vi "PointGrey Grasshopper_Settings.vi"(9 "Which cameras record":bool[](array[boolean]), 10 "Camera to address":i32 min=0 max=0 step=1, 11 "Camera References":T1[](array[typedef])) -> (1 "Which cameras record out":bool[](array[boolean]))   [LabVIEW 2015]
uses:
  <vilib>/userdefined/High Color/IMAQdx.ctl
  <vilib>/vision/driver/IMAQdx.llb/IMAQdx Attribute Visibility.ctl
  <vilib>/Utility/miscctls.llb/LVOutOfRangeActionTypeDef.ctl
  <vilib>/vision/driver/NI_Vision_Acquisition_Software.lvlib
  <resource>/objmgr/imaqdx.rc
panel:
  in  "CameraCommand":string
  in  "CameraEnum":u16(ring) items=["Off", "Once", "Continuous"]
  in  "CameraBool":bool
  in  "CameraString":string
  in  "CameraDBL":dbl
  in  "CameraI64":i64
  in  "CameraU32":u32
  in  "Tree":string(tree)
  in  "OK Button":bool
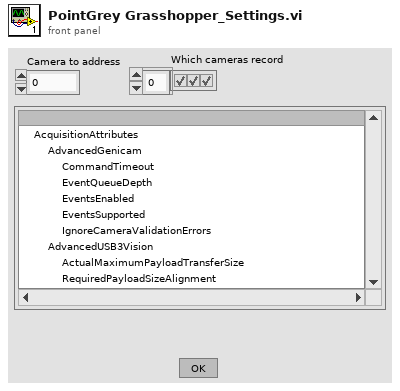
[diagram p1: front panel]
types:
  T1 = typedef "IMAQdx.ctl" = refnum<k21>
  T2 = typedef "LVOutOfRangeActionTypeDef.ctl" = cluster{"Out of Range Action Minimum":u8, "Out of Range Action Maximum":u8, "Out of Range Action Increment":u8}
  T3 = typedef "NI_Vision_Acquisition_Software.lvlib/IMAQdx Attribute Visibility.ctl" = enum32{"Simple", "Intermediate", "Advanced"}
  T4 = enum8{"Enabled", "Disabled", "Disabled and Grayed Out"}
  T5 = typedef "NI_Vision_Acquisition_Software.lvlib/IMAQdx Attribute Type.ctl" = enum32{"U32", "I64", "DBL", "String", "Enum", "Bool", "Command"}
  T6 = cluster{"Attribute Type":T5, "Readable":bool, "Writable":bool, "Attribute Name":string}[]
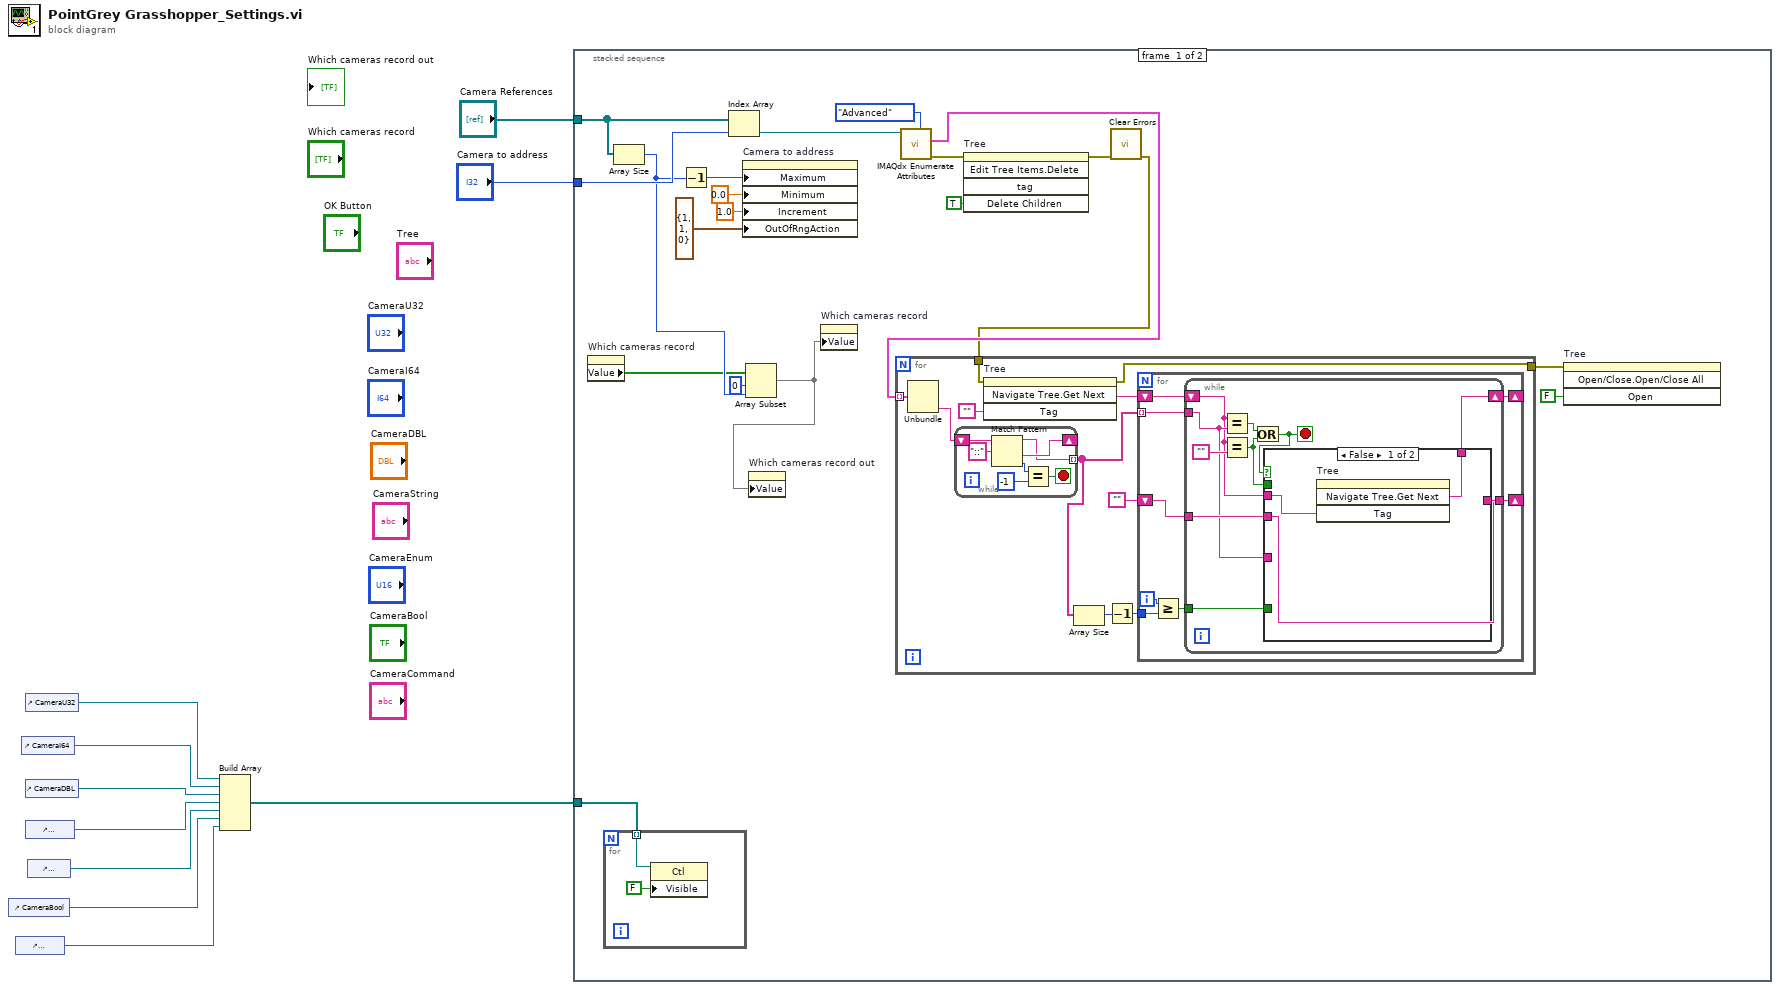
[diagram p0: block diagram]
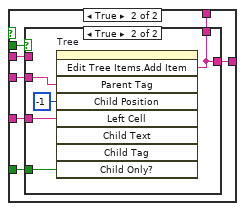
[diagram p2: hidden frame]
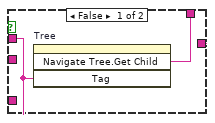
[diagram p3: hidden frame]
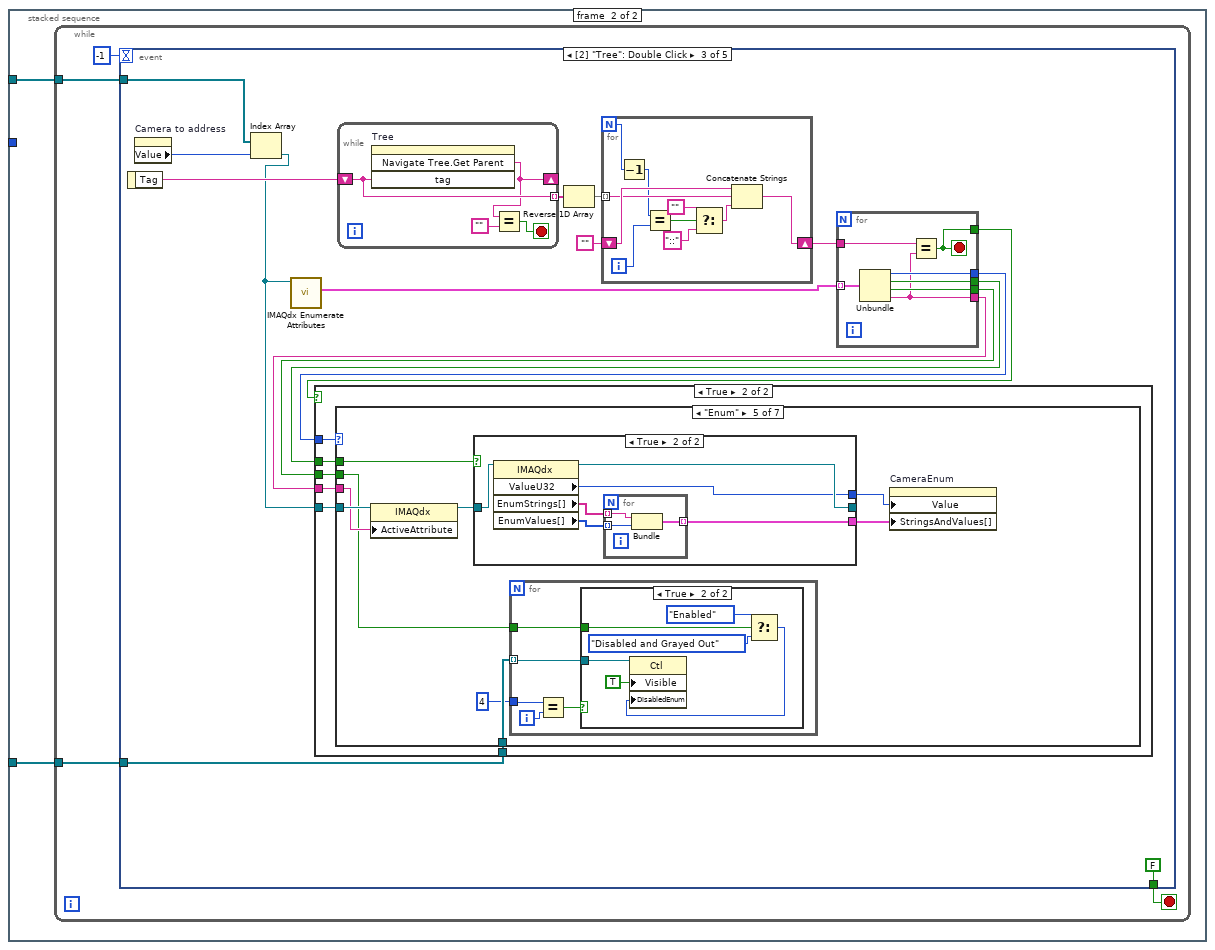
[diagram p4: hidden frame]
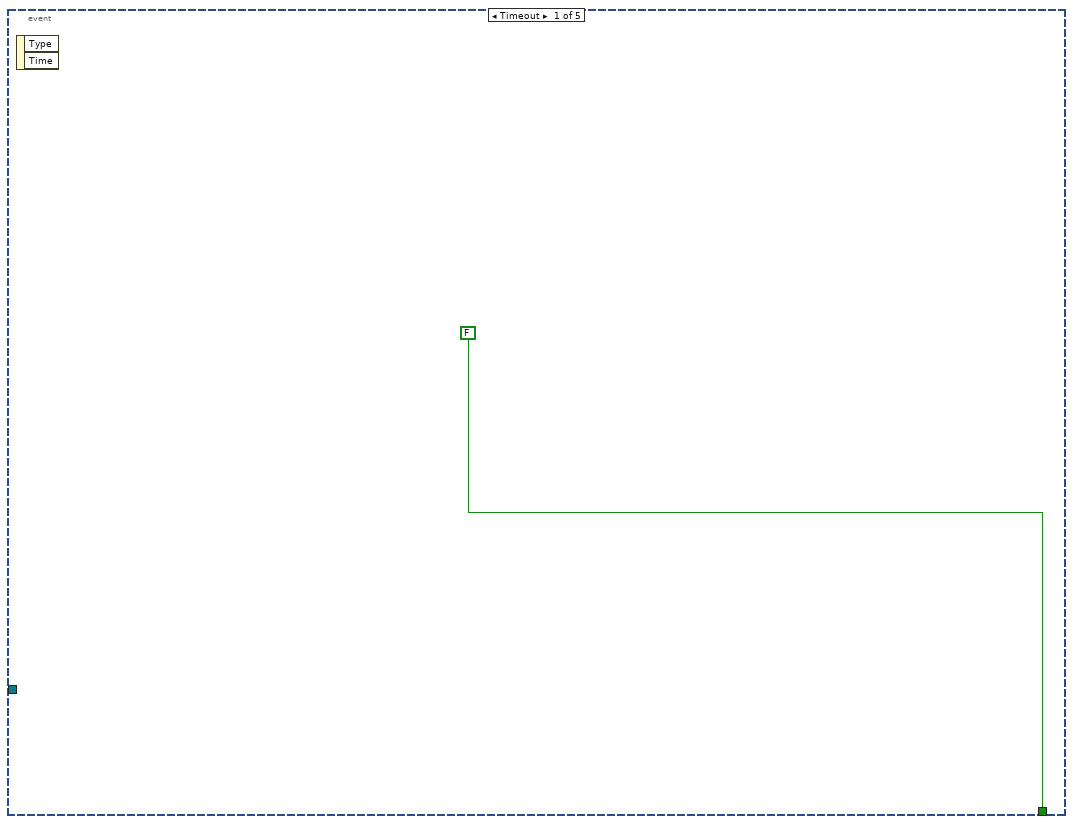
[diagram p5: hidden frame]
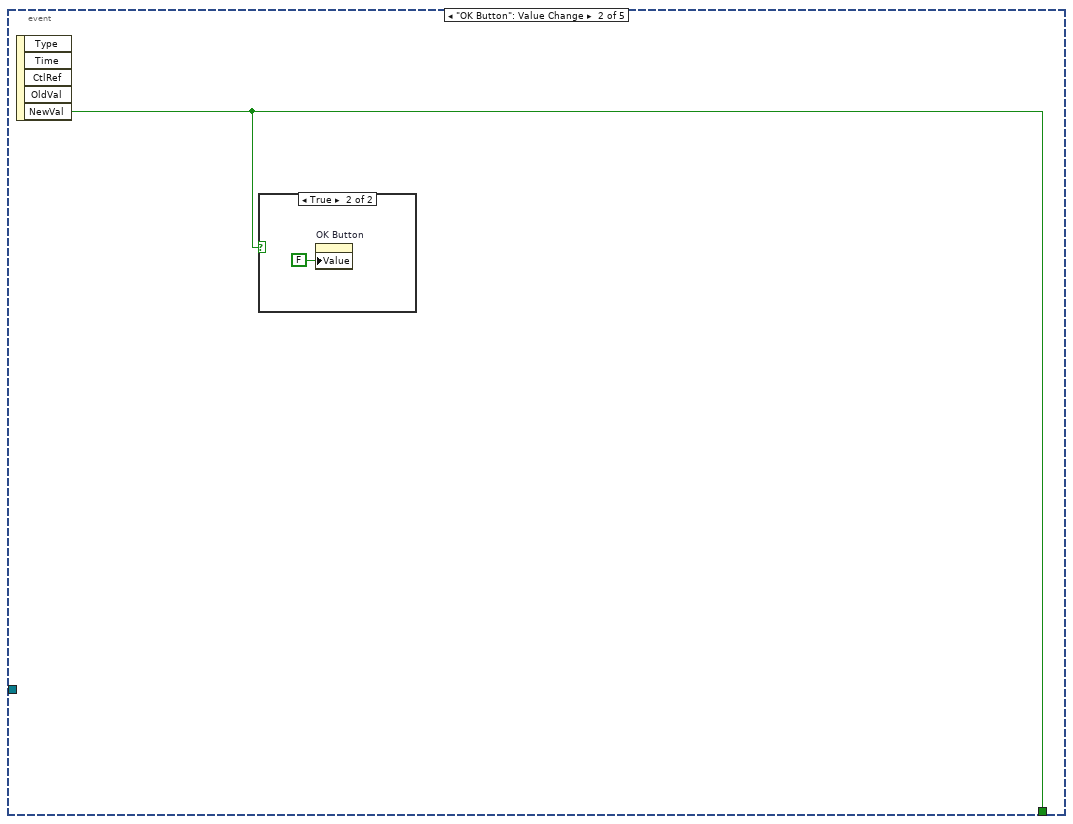
[diagram p6: hidden frame]
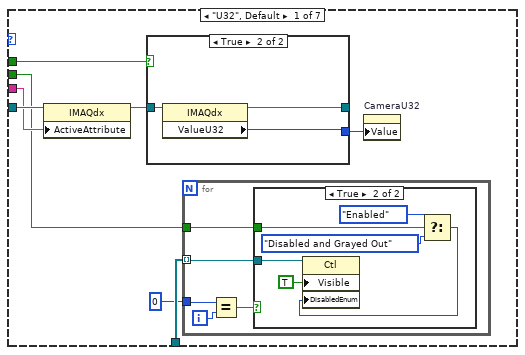
[diagram p9: hidden frame]
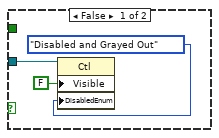
[diagram p10: hidden frame]
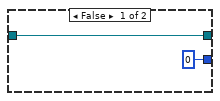
[diagram p11: hidden frame]
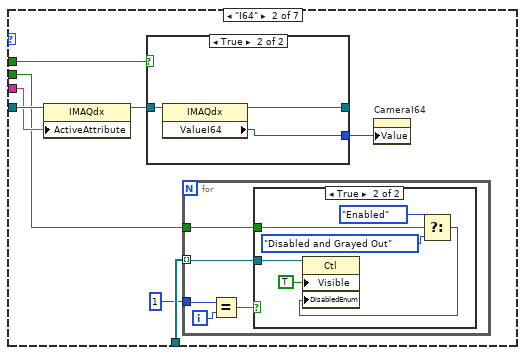
[diagram p12: hidden frame]
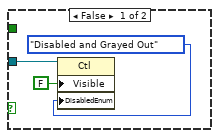
[diagram p13: hidden frame]
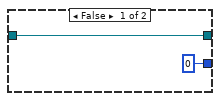
[diagram p14: hidden frame]
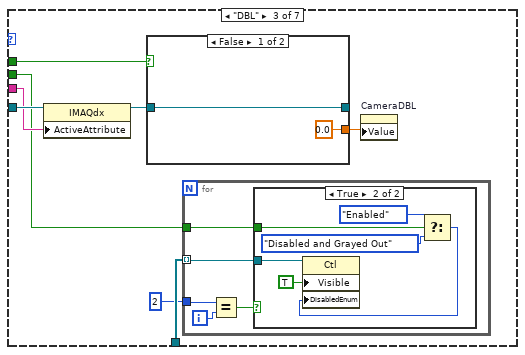
[diagram p15: hidden frame]
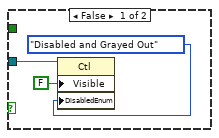
[diagram p16: hidden frame]
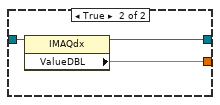
[diagram p17: hidden frame]
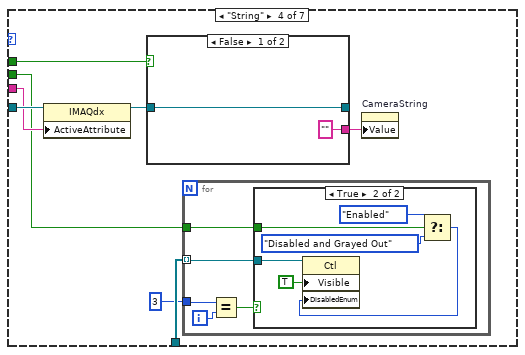
[diagram p18: hidden frame]
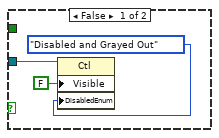
[diagram p19: hidden frame]
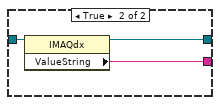
[diagram p20: hidden frame]
diagram:
  n1 = control-ref of="CameraBool"() -> (w3:refnum<vi>)
  n2 = control-ref of="CameraCommand"() -> (w2:refnum<vi>)
  n3 = control-ref of="CameraI64"() -> (w7:refnum<vi>)
  n4 = control-ref of="CameraU32"() -> (w8:refnum<vi>)
  n5 = control-ref of="CameraDBL"() -> (w6:refnum<vi>)
  n6 = control-ref of="CameraString"() -> (w5:refnum<vi>)
  n7 = control-ref of="CameraEnum"() -> (w4:refnum<vi>)
  n8 = Build Array(w8, w7, w6, w5, w4, w3, w2) -> (w1:refnum<vi>[])
  n9 = stacked-sequence {
    tunnel: "Camera References" -> [w19 w86]
    tunnel: "Camera to address" -> [w21 _]
    tunnel: w1 -> [w20 w85]
    frame #0 {
      n10 = property on="Which cameras record" class="Arr (strict)"() -> ("Value"=w12:bool[])  [unwired: 2 in, 2 out]
      n11 = for {
        tunnel: w20 -> [w32] mode=indexing
        n12 = property class="Ctl"(reference=w32, "Visible"=FALSE) -> ()  [unwired: 1 in, 2 out]
      }
      n13 = Array Size(array=w19) -> (size(s)=w14:i32)
      n14 = Decrement(x=w14) -> (x-1=w15:i32)
      n15 = Index Array(array=w19, index=w21) -> (element=w22:T1)
      n16 = property on="Camera to address" class="DigNum (strict)"("Maximum"=w15, "Minimum"=0.0 ("Data Entry Limits:Minimum"), "Increment"=1.0 ("Data Entry Limits:Increment"), "OutOfRngAction"=T2 {"Out of Range Action Minimum"=1, "Out of Range Action Maximum"=1, "Out of Range Action Increment"=0} ("Response to Value Outside Limits")) -> ()  [unwired: 2 in, 2 out]
      n17 = Array Subset(array=w12, index=0, length=w14) -> (w11:bool[])
      n18 = property on="Which cameras record out" class="Arr (strict)"("Value"=w11) -> ()  [unwired: 2 in, 2 out]
      n19 = property on="Which cameras record" class="Arr (strict)"("Value"=w11) -> ()  [unwired: 2 in, 2 out]
      n20 = call <vilib>:"IMAQdx Enumerate Attributes.vi"("Visibility"=IMAQdx_Attribute_Visibility."Advanced", "Session In"=w22) -> ("error out"=w26:errorcluster, "Attribute Information Array"=w30:T6)  [unwired: 7 in, 1 out]
      n21 = invoke on="Tree" class="Tree (strict)" method="Edit Tree Items.Delete"(error in=w26, "Delete Children"=TRUE ("Delete Children?")) -> (error out=w25:errorcluster)  [unwired: 3 in, 4 out]
      n22 = call <vilib>:"Clear Errors.vi"("error in (no error)"=w25) -> ("error out"=w27:errorcluster)  [unwired: 5 in, 1 out]
      n23 = for {
        tunnel: w30 -> [w42] mode=indexing
        tunnel: w27 -> [w34]
        tunnel: [w33] -> w29
        n24 = Unbundle(w42) -> ("Attribute Name"=w41:string)  [unwired: 3 out]
        n25 = while {
          shift-right: [w82] -> _
          shift-left: w41 -> [w84]
          tunnel: [w78] -> w38 mode=indexing
          stop <- w79 stop-if-true
          n26 = Match Pattern(string=w84, regular expression="::") -> (before substring=w78:string, after substring=w82:string, offset past match=w81:i32)  [unwired: 1 in, 1 out]
          n27 = Equal?(x=w81, y=-1) -> (x = y?=w79:bool)
        }
        n28 = invoke on="Tree" class="Tree (strict)" method="Navigate Tree.Get Next"(error in=w34, "Tag"="") -> (error out=w33:errorcluster, "Navigate Tree:Get Next Item"=w36:string)  [unwired: 2 in, 2 out]
        n29 = Array Size(array=w38) -> (size(s)=w39:i32)
        n30 = Decrement(x=w39) -> (x-1=w35:i32)
        n31 = for {
          tunnel: w38 -> [w50] mode=indexing
          shift-right: [w49] -> _
          shift-left: "" -> [w48]
          tunnel: w35 -> [w46]
          shift-right: [w43] -> _
          shift-left: w36 -> [w44]
          i -> [w45]
          n32 = Greater Or Equal?(x=w45, y=w46) -> (x >= y?=w47:bool)
          n33 = while {
            shift-right: [w51] -> w43
            shift-left: w44 -> [w52]
            tunnel: w50 -> [w53]
            tunnel: [w56] -> w49
            tunnel: w48 -> [w55]
            tunnel: w47 -> [w54]
            stop <- w58 stop-if-true
            n34 = Equal?(x=w52, y=w53) -> (x = y?=w59:bool)
            n35 = Equal?(x=w52, y="") -> (x = y?=w57:bool)
            n36 = Or(x=w59, y=w57) -> (x .or. y?=w58:bool)
            n37 = case shown="False" w58 {
              tunnel: w52 -> [w62 w69]
              tunnel: w57 -> [_ w70]
              tunnel: [w63 w68] -> w56
              tunnel: w55 -> [w63 w67]
              tunnel: w54 -> [_ w66]
              tunnel: w53 -> [_ w65]
              tunnel: [w61 w64] -> w51
              frame False {
                n38 = invoke on="Tree" class="Tree (strict)" method="Navigate Tree.Get Next"("Tag"=w62) -> ("Navigate Tree:Get Next Item"=w61:string)  [unwired: 3 in, 3 out]
              }
              frame True {
                n39 = case shown="True" w70 {
                  tunnel: w69 -> [w71 _]
                  tunnel: [w71 w73] -> w68
                  tunnel: w67 -> [_ w74]
                  tunnel: w66 -> [_ w76]
                  tunnel: w65 -> [_ w75]
                  tunnel: [w72 w73] -> w64
                  frame False {
                    n40 = invoke on="Tree" class="Tree (strict)" method="Navigate Tree.Get Child"("Tag"=w71) -> ("Navigate Tree:Get Child"=w72:string)  [unwired: 3 in, 3 out]
                  }
                  frame True {
                    n41 = invoke on="Tree" class="Tree (strict)" method="Edit Tree Items.Add Item"("Parent Tag"=w74, "Child Position"=-1, "Left Cell"=w75, "Child Only?"=w76) -> ("Edit Tree Items:Add Item"=w73:string)  [unwired: 5 in, 8 out]
                  }
                }
              }
            }
          }
        }
      }
      n42 = invoke on="Tree" class="Tree (strict)" method="Open/Close.Open/Close All"(error in=w29, "Open"=FALSE ("Open?")) -> ()  [unwired: 2 in, 4 out]
    }
    frame #1 {
      n43 = while {
        tunnel: w86 -> [w88]
        tunnel: w85 -> [w87]
        stop <- w89 stop-if-true
        n44 = event shown="[2] \"Tree\": Double Click" {
          selector: _ -> [_ _ _ _ _]
          dyn-events: _ -> [_ _ _ _ _]
          timeout: -1 -> [_ _ _ _ _]
          tunnel: [FALSE ("NewVal") w92 FALSE ("NewVal") FALSE ("NewVal") FALSE ("NewVal")] -> w89
          tunnel: w88 -> [_ _ w98 w338 w343]
          tunnel: w87 -> [_ _ w95 _ w345]
          event Timeout {
            n45 = event-data() -> ()  [unwired: 1 in, 2 out]
          }
          event "OK Button": Value Change {
            n46 = event-data() -> ("NewVal"=w92:bool)  [unwired: 1 in, 4 out]
            n47 = case shown="True" w92 {
              frame False {
              }
              frame True {
                n48 = property on="OK Button" class="Bool (strict)"("Value"=FALSE ("OK Button")) -> ()  [unwired: 2 in, 2 out]
              }
            }
          }
          event "Tree": Double Click {
            n49 = event-data() -> ("Tag"=w99:string)  [unwired: 1 in]
            n50 = property on="Camera to address" class="DigNum (strict)"() -> ("Value"=w97:i32)  [unwired: 2 in, 2 out]
            n51 = Index Array(array=w98, index=w97) -> (element=w96:T1)
            n52 = call <vilib>:"IMAQdx Enumerate Attributes.vi"("Session In"=w96) -> ("Attribute Information Array"=w100:T6)  [unwired: 8 in, 2 out]
            n53 = while {
              shift-right: [w322] -> _
              shift-left: w99 -> [w323]
              tunnel: [w323] -> w109 mode=indexing
              stop <- w320 stop-if-true
              n54 = invoke on="Tree" class="Tree (strict)" method="Navigate Tree.Get Parent"("tag"=w323) -> ("Navigate Tree:Get Parent"=w322:string)  [unwired: 3 in, 3 out]
              n55 = Equal?(x=w322, y="") -> (x = y?=w320:bool)
            }
            n56 = Reverse 1D Array(array=w109) -> (reversed array=w107:string[])
            n57 = for {
              N -> [w330]
              tunnel: w107 -> [w332] mode=indexing
              shift-right: [w324] -> w106
              shift-left: "" -> [w333]
              i -> [w327]
              n58 = Decrement(x=w330) -> (x-1=w328:i32)
              n59 = Equal?(x=w328, y=w327) -> (x = y?=w329:bool)
              n60 = Select(t="", s=w329, f="::" ("t")) -> (s? t:f=w331:string)
              n61 = Concatenate Strings(w333, w332, w331) -> (w324:string)
            }
            n62 = for {
              tunnel: w100 -> [w319] mode=indexing
              tunnel: w106 -> [w318]
              tunnel: [w317] -> w102
              tunnel: [w316] -> w103
              tunnel: [w315] -> w104
              tunnel: [w314] -> w105
              tunnel: [w313] -> w101
              stop <- w314 stop-if-true
              n63 = Unbundle(w319) -> ("Attribute Type"=w315:T5, "Readable"=w316:bool, "Writable"=w317:bool, "Attribute Name"=w313:string)
              n64 = Equal?(x=w318, y=w313) -> (x = y?=w314:bool)
            }
            n65 = case shown="True" w105 {
              tunnel: w104 -> [_ w115]
              tunnel: w103 -> [_ w114]
              tunnel: w102 -> [_ w113]
              tunnel: w101 -> [_ w112]
              tunnel: w96 -> [_ w111]
              tunnel: w95 -> [_ w110]
              frame False {
              }
              frame True {
                n66 = case shown="\"Enum\"" w115 {
                  tunnel: w114 -> [w117 w144 w171 w198 w225 w260 w287]
                  tunnel: w113 -> [w116 w143 w170 w197 w224 w259 w286]
                  tunnel: w112 -> [w122 w149 w176 w203 w231 w265 w292]
                  tunnel: w111 -> [w123 w150 w177 w204 w232 w266 w293]
                  tunnel: w110 -> [w120 w147 w174 w201 w229 w263 w290]
                  frame "U32", Default {
                    n67 = property class="IMAQdx"(reference=w123, "ActiveAttribute"=w122) -> (reference out=w121:T1)  [unwired: 1 in, 1 out]
                    n68 = case shown="True" w117 {
                      tunnel: w121 -> [w139 w142]
                      tunnel: [w139 w141] -> _
                      tunnel: [u32 0 ("ValueU32") w140] -> w118
                      frame False {
                      }
                      frame True {
                        n69 = property class="IMAQdx"(reference=w142) -> (reference out=w141:T1, "ValueU32"=w140:u32)  [unwired: 1 in, 1 out]
                      }
                    }
                    n70 = for {
                      tunnel: w120 -> [w128] mode=indexing
                      tunnel: 0 -> [w125]
                      tunnel: w116 -> [w124]
                      i -> [w127]
                      n71 = Equal?(x=w125, y=w127) -> (x = y?=w126:bool)
                      n72 = case shown="True" w126 {
                        tunnel: w128 -> [w131 w137]
                        tunnel: w124 -> [_ w135]
                        frame False {
                          n73 = property class="Ctl"(reference=w131, "Visible"=FALSE, "DisabledEnum"=T4."Disabled and Grayed Out" ("Disabled")) -> ()  [unwired: 1 in, 2 out]
                        }
                        frame True {
                          n74 = Select(t=T4."Enabled" ("Disabled"), s=w135, f=T4."Disabled and Grayed Out" ("Disabled")) -> (s? t:f=w132:T4)
                          n75 = property class="Ctl"(reference=w137, "Visible"=TRUE, "DisabledEnum"=w132) -> ()  [unwired: 1 in, 2 out]
                        }
                      }
                    }
                    n76 = property on="CameraU32" class="DigNum (strict)"("Value"=w118) -> ()  [unwired: 2 in, 2 out]
                  }
                  frame "I64" {
                    n77 = property class="IMAQdx"(reference=w150, "ActiveAttribute"=w149) -> (reference out=w148:T1)  [unwired: 1 in, 1 out]
                    n78 = case shown="True" w144 {
                      tunnel: w148 -> [w166 w169]
                      tunnel: [w166 w168] -> _
                      tunnel: [i64 0 ("ValueI64") w167] -> w145
                      frame False {
                      }
                      frame True {
                        n79 = property class="IMAQdx"(reference=w169) -> (reference out=w168:T1, "ValueI64"=w167:i64)  [unwired: 1 in, 1 out]
                      }
                    }
                    n80 = for {
                      tunnel: w147 -> [w155] mode=indexing
                      tunnel: 1 -> [w152]
                      tunnel: w143 -> [w151]
                      i -> [w154]
                      n81 = Equal?(x=w152, y=w154) -> (x = y?=w153:bool)
                      n82 = case shown="True" w153 {
                        tunnel: w155 -> [w158 w164]
                        tunnel: w151 -> [_ w162]
                        frame False {
                          n83 = property class="Ctl"(reference=w158, "Visible"=FALSE, "DisabledEnum"=T4."Disabled and Grayed Out" ("Disabled")) -> ()  [unwired: 1 in, 2 out]
                        }
                        frame True {
                          n84 = Select(t=T4."Enabled" ("Disabled"), s=w162, f=T4."Disabled and Grayed Out" ("Disabled")) -> (s? t:f=w159:T4)
                          n85 = property class="Ctl"(reference=w164, "Visible"=TRUE, "DisabledEnum"=w159) -> ()  [unwired: 1 in, 2 out]
                        }
                      }
                    }
                    n86 = property on="CameraI64" class="DigNum (strict)"("Value"=w145) -> ()  [unwired: 2 in, 2 out]
                  }
                  frame "DBL" {
                    n87 = property class="IMAQdx"(reference=w177, "ActiveAttribute"=w176) -> (reference out=w175:T1)  [unwired: 1 in, 1 out]
                    n88 = case shown="False" w171 {
                      tunnel: w175 -> [w193 w196]
                      tunnel: [w193 w195] -> _
                      tunnel: [0.0 ("ValueDBL") w194] -> w172
                      frame False {
                      }
                      frame True {
                        n89 = property class="IMAQdx"(reference=w196) -> (reference out=w195:T1, "ValueDBL"=w194:dbl)  [unwired: 1 in, 1 out]
                      }
                    }
                    n90 = for {
                      tunnel: w174 -> [w182] mode=indexing
                      tunnel: 2 -> [w179]
                      tunnel: w170 -> [w178]
                      i -> [w181]
                      n91 = Equal?(x=w179, y=w181) -> (x = y?=w180:bool)
                      n92 = case shown="True" w180 {
                        tunnel: w182 -> [w185 w191]
                        tunnel: w178 -> [_ w189]
                        frame False {
                          n93 = property class="Ctl"(reference=w185, "Visible"=FALSE, "DisabledEnum"=T4."Disabled and Grayed Out" ("Disabled")) -> ()  [unwired: 1 in, 2 out]
                        }
                        frame True {
                          n94 = Select(t=T4."Enabled" ("Disabled"), s=w189, f=T4."Disabled and Grayed Out" ("Disabled")) -> (s? t:f=w186:T4)
                          n95 = property class="Ctl"(reference=w191, "Visible"=TRUE, "DisabledEnum"=w186) -> ()  [unwired: 1 in, 2 out]
                        }
                      }
                    }
                    n96 = property on="CameraDBL" class="DigNum (strict)"("Value"=w172) -> ()  [unwired: 2 in, 2 out]
                  }
                  frame "String" {
                    n97 = property class="IMAQdx"(reference=w204, "ActiveAttribute"=w203) -> (reference out=w202:T1)  [unwired: 1 in, 1 out]
                    n98 = case shown="False" w198 {
                      tunnel: w202 -> [w220 w223]
                      tunnel: [w220 w222] -> _
                      tunnel: ["" ("ValueString") w221] -> w199
                      frame False {
                      }
                      frame True {
                        n99 = property class="IMAQdx"(reference=w223) -> (reference out=w222:T1, "ValueString"=w221:string)  [unwired: 1 in, 1 out]
                      }
                    }
                    n100 = for {
                      tunnel: w201 -> [w209] mode=indexing
                      tunnel: 3 -> [w206]
                      tunnel: w197 -> [w205]
                      i -> [w208]
                      n101 = Equal?(x=w206, y=w208) -> (x = y?=w207:bool)
                      n102 = case shown="True" w207 {
                        tunnel: w209 -> [w212 w218]
                        tunnel: w205 -> [_ w216]
                        frame False {
                          n103 = property class="Ctl"(reference=w212, "Visible"=FALSE, "DisabledEnum"=T4."Disabled and Grayed Out" ("Disabled")) -> ()  [unwired: 1 in, 2 out]
                        }
                        frame True {
                          n104 = Select(t=T4."Enabled" ("Disabled"), s=w216, f=T4."Disabled and Grayed Out" ("Disabled")) -> (s? t:f=w213:T4)
                          n105 = property class="Ctl"(reference=w218, "Visible"=TRUE, "DisabledEnum"=w213) -> ()  [unwired: 1 in, 2 out]
                        }
                      }
                    }
                    n106 = property on="CameraString" class="Str"("Value"=w199) -> ()  [unwired: 2 in, 2 out]
                  }
                  frame "Enum" {
                    n107 = property class="IMAQdx"(reference=w232, "ActiveAttribute"=w231) -> (reference out=w230:T1)  [unwired: 1 in, 1 out]
                    n108 = case shown="True" w225 {
                      tunnel: w230 -> [w249 w255]
                      tunnel: [w249 w254] -> _
                      tunnel: [u32 0 ("ValueU32") w251] -> w227
                      tunnel: [cluster{string, u32}[] [] w250] -> w226
                      frame False {
                      }
                      frame True {
                        n109 = property class="IMAQdx"(reference=w255) -> (reference out=w254:T1, "ValueU32"=w251:u32, "EnumStrings[]"=w253:string[], "EnumValues[]"=w252:u32[])  [unwired: 1 in, 1 out]
                        n110 = for {
                          tunnel: w253 -> [w257] mode=indexing
                          tunnel: w252 -> [w258] mode=indexing
                          tunnel: [w256] -> w250 mode=indexing
                          n111 = Bundle(w257, w258) -> (w256:cluster{string, u32})  [unwired: 1 in]
                        }
                      }
                    }
                    n112 = for {
                      tunnel: w229 -> [w237] mode=indexing
                      tunnel: 4 -> [w234]
                      tunnel: w224 -> [w233]
                      i -> [w236]
                      n113 = Equal?(x=w234, y=w236) -> (x = y?=w235:bool)
                      n114 = case shown="True" w235 {
                        tunnel: w237 -> [w240 w246]
                        tunnel: w233 -> [_ w244]
                        frame False {
                          n115 = property class="Ctl"(reference=w240, "Visible"=FALSE, "DisabledEnum"=T4."Disabled and Grayed Out" ("Disabled")) -> ()  [unwired: 1 in, 2 out]
                        }
                        frame True {
                          n116 = Select(t=T4."Enabled" ("Disabled"), s=w244, f=T4."Disabled and Grayed Out" ("Disabled")) -> (s? t:f=w241:T4)
                          n117 = property class="Ctl"(reference=w246, "Visible"=TRUE, "DisabledEnum"=w241) -> ()  [unwired: 1 in, 2 out]
                        }
                      }
                    }
                    n118 = property on="CameraEnum" class="Ring (strict)"("Value"=w227, "StringsAndValues[]"=w226) -> ()  [unwired: 2 in, 2 out]
                  }
                  frame "Bool" {
                    n119 = property class="IMAQdx"(reference=w266, "ActiveAttribute"=w265) -> (reference out=w264:T1)  [unwired: 1 in, 1 out]
                    n120 = case shown="False" w260 {
                      tunnel: w264 -> [w282 w285]
                      tunnel: [w282 w284] -> _
                      tunnel: [FALSE ("ValueBool") w283] -> w261
                      frame False {
                      }
                      frame True {
                        n121 = property class="IMAQdx"(reference=w285) -> (reference out=w284:T1, "ValueBool"=w283:bool)  [unwired: 1 in, 1 out]
                      }
                    }
                    n122 = for {
                      tunnel: w263 -> [w271] mode=indexing
                      tunnel: 5 -> [w268]
                      tunnel: w259 -> [w267]
                      i -> [w270]
                      n123 = Equal?(x=w268, y=w270) -> (x = y?=w269:bool)
                      n124 = case shown="True" w269 {
                        tunnel: w271 -> [w274 w280]
                        tunnel: w267 -> [_ w278]
                        frame False {
                          n125 = property class="Ctl"(reference=w274, "Visible"=FALSE, "DisabledEnum"=T4."Disabled and Grayed Out" ("Disabled")) -> ()  [unwired: 1 in, 2 out]
                        }
                        frame True {
                          n126 = Select(t=T4."Enabled" ("Disabled"), s=w278, f=T4."Disabled and Grayed Out" ("Disabled")) -> (s? t:f=w275:T4)
                          n127 = property class="Ctl"(reference=w280, "Visible"=TRUE, "DisabledEnum"=w275) -> ()  [unwired: 1 in, 2 out]
                        }
                      }
                    }
                    n128 = property on="CameraBool" class="Bool (strict)"("Value"=w261) -> ()  [unwired: 2 in, 2 out]
                  }
                  frame "Command" {
                    n129 = property class="IMAQdx"(reference=w293, "ActiveAttribute"=w292) -> (reference out=w291:T1)  [unwired: 1 in, 1 out]
                    n130 = case shown="True" w287 {
                      tunnel: w291 -> [w309 w312]
                      tunnel: [w309 w311] -> _
                      tunnel: ["" ("ValueString") w310] -> w288
                      frame False {
                      }
                      frame True {
                        n131 = property class="IMAQdx"(reference=w312) -> (reference out=w311:T1, "ValueString"=w310:string)  [unwired: 1 in, 1 out]
                      }
                    }
                    n132 = for {
                      tunnel: w290 -> [w298] mode=indexing
                      tunnel: 6 -> [w295]
                      tunnel: w286 -> [w294]
                      i -> [w297]
                      n133 = Equal?(x=w295, y=w297) -> (x = y?=w296:bool)
                      n134 = case shown="True" w296 {
                        tunnel: w298 -> [w301 w307]
                        tunnel: w294 -> [_ w305]
                        frame False {
                          n135 = property class="Ctl"(reference=w301, "Visible"=FALSE, "DisabledEnum"=T4."Disabled and Grayed Out" ("Disabled")) -> ()  [unwired: 1 in, 2 out]
                        }
                        frame True {
                          n136 = Select(t=T4."Enabled" ("Disabled"), s=w305, f=T4."Disabled and Grayed Out" ("Disabled")) -> (s? t:f=w302:T4)
                          n137 = property class="Ctl"(reference=w307, "Visible"=TRUE, "DisabledEnum"=w302) -> ()  [unwired: 1 in, 2 out]
                        }
                      }
                    }
                    n138 = property on="CameraCommand" class="Str"("Value"=w288) -> ()  [unwired: 2 in, 2 out]
                  }
                }
              }
            }
          }
          event "Which cameras record": Value Change {
            n139 = event-data() -> ("NewVal"=w336:bool[])  [unwired: 1 in]
            n140 = Array Size(array=w338) -> (size(s)=w337:i32)
            n141 = Array Subset(array=w336, index=0, length=w337) -> (w334:bool[])
            n142 = property on="Which cameras record" class="Arr (strict)"("Value"=w334) -> ()  [unwired: 2 in, 2 out]
            n143 = property on="Which cameras record out" class="Arr (strict)"("Value"=w334) -> ()  [unwired: 2 in, 2 out]
          }
          event "CameraU32", "CameraI64", "CameraDBL", "CameraString", "CameraBool", "CameraEnum", "CameraCommand": Value Change {
            n144 = event-data() -> ("CtlRef"=w344:refnum<vi>, "NewVal"=w346:variant)  [unwired: 1 in]
            n145 = property on="Camera to address" class="DigNum (strict)"() -> ("Value"=w341:i32)  [unwired: 2 in, 2 out]
            n146 = Index Array(array=w343, index=w341) -> (element=w342:T1)
            n147 = for {
              tunnel: w345 -> [w351] mode=indexing
              tunnel: w344 -> [w350]
              tunnel: [w348] -> w347
              i -> [w348]
              stop <- w349 stop-if-true
              n148 = Equal?(x=w350, y=w351) -> (x = y?=w349:bool)
            }
            n149 = case shown="0, Default" w347 {
              tunnel: w346 -> [w355 w359 w363 w367 w371 w375 w379]
              tunnel: w342 -> [w354 w358 w362 w366 w370 w374 w378]
              frame 0, Default {
                n150 = Variant To Data(type=u32 0, Variant=w355) -> (data=w353:u32)  [unwired: 1 in, 1 out]
                n151 = property class="IMAQdx"(reference=w354, "ValueU32"=w353) -> ()  [unwired: 1 in, 2 out]
              }
              frame 1 {
                n152 = Variant To Data(type=i64 0, Variant=w359) -> (data=w357:i64)  [unwired: 1 in, 1 out]
                n153 = property class="IMAQdx"(reference=w358, "ValueI64"=w357) -> ()  [unwired: 1 in, 2 out]
              }
              frame 2 {
                n154 = Variant To Data(type=0.0, Variant=w363) -> (data=w361:dbl)  [unwired: 1 in, 1 out]
                n155 = property class="IMAQdx"(reference=w362, "ValueDBL"=w361) -> ()  [unwired: 1 in, 2 out]
              }
              frame 3 {
                n156 = Variant To Data(type="", Variant=w367) -> (data=w365:string)  [unwired: 1 in, 1 out]
                n157 = property class="IMAQdx"(reference=w366, "ValueString"=w365) -> ()  [unwired: 1 in, 2 out]
              }
              frame 4 {
                n158 = Variant To Data(type=u32 0, Variant=w371) -> (data=w369:u32)  [unwired: 1 in, 1 out]
                n159 = property class="IMAQdx"(reference=w370, "ValueU32"=w369) -> ()  [unwired: 1 in, 2 out]
              }
              frame 5 {
                n160 = Variant To Data(type=TRUE, Variant=w375) -> (data=w373:bool)  [unwired: 1 in, 1 out]
                n161 = property class="IMAQdx"(reference=w374, "ValueBool"=w373) -> ()  [unwired: 1 in, 2 out]
              }
              frame 6 {
                n162 = Variant To Data(type="", Variant=w379) -> (data=w377:string)  [unwired: 1 in, 1 out]
                n163 = property class="IMAQdx"(reference=w378, "ValueString"=w377) -> ()  [unwired: 1 in, 2 out]
              }
            }
          }
        }
      }
    }
  }
